vi "flip_switch.vi"(0 "PrepLineObject.lvclass":refnum<class "PrepLineObject.lvclass">, 3 "error in (no error)":errorcluster) -> (7 "PrepLineObject out":refnum<class "PrepLineObject.lvclass">, 10 "error out":errorcluster)   [LabVIEW 2017]
doc: "The switch that belongs to the \"PrepLineObject\" is being switched to the state as given in the private property."
uses:
  Classes/PrepLineObject/PrepLineObject.lvclass
  global variables.vi
  Classes/Instrument/instrument.lvclass
  Classes/StatusLog/StatusLog.lvclass
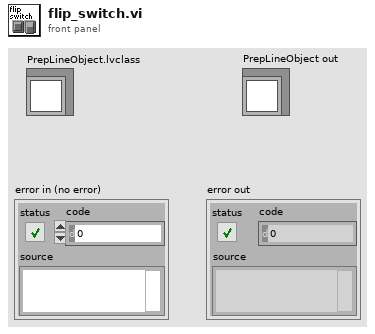
[diagram p1: front panel]
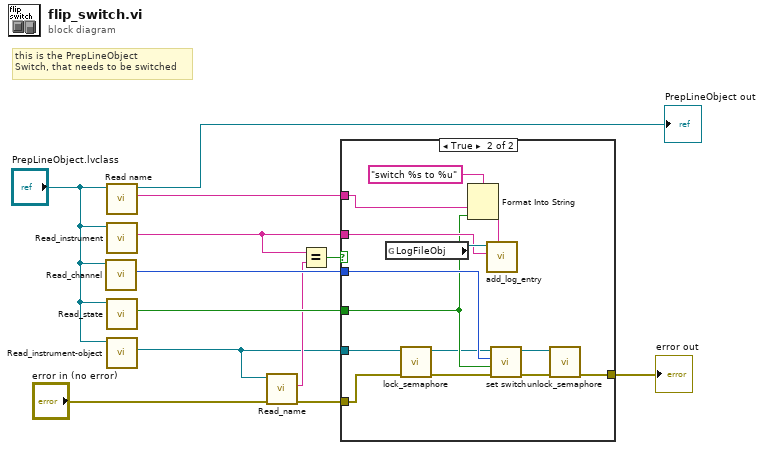
[diagram p0: block diagram]
diagram:
  # "this is the PrepLineObject\nSwitch, that needs to be switched"
  n1 = call-dynamic "Read_channel.vi"("PrepLineObject in"="PrepLineObject.lvclass") -> ("channel"=w7:u16)  [unwired: 8 in, 2 out]
  n2 = call-dynamic "Read name.vi"("PrepLineObject in"="PrepLineObject.lvclass") -> ("name"=w9:string, "PrepLineObject out"=→"PrepLineObject out":refnum<class "PrepLineObject.lvclass">)  [unwired: 8 in, 1 out]
  n3 = call-dynamic "Read_instrument.vi"("PrepLinePictureObjects in"="PrepLineObject.lvclass") -> ("instrument name"=w8:string)  [unwired: 7 in, 2 out]
  n4 = call-dynamic "Read_state.vi"("PrepLineObject in"="PrepLineObject.lvclass") -> ("state"=w6:bool)  [unwired: 8 in, 2 out]
  n5 = call-dynamic "Read_instrument-object.vi"("PrepLineObject in"="PrepLineObject.lvclass") -> ("instrument.lvclass"=w1:refnum<class "instrument.lvclass">)  [unwired: 8 in, 2 out]
  n6 = call-dynamic "Read_name.vi"("error in (no error)"="error in (no error)", "instrument in"=w1) -> ("error out"=w2:errorcluster, "name"=w4:string)  [unwired: 7 in, 1 out]
  n7 = Equal?(x=w8, y=w4) -> (x = y?=w3:bool)
  n8 = case shown="True" w3 {
    tunnel: w1 -> [_ w20]
    tunnel: w7 -> [_ w27]
    tunnel: w6 -> [_ w21]
    tunnel: w2 -> [w13 w19]
    tunnel: [w13 w14] -> w11
    tunnel: w9 -> [_ w22]
    tunnel: w8 -> [_ w23]
    frame False {
      # "wrong instrument"
    }
    frame True {
      n9 = global read "global variables.vi" "LogFileObj"() -> (w26:refnum<class "StatusLog.lvclass">)
      n10 = call-dynamic "lock_semaphore.vi"("error in (no error)"=w19, "instrument in"=w20) -> ("error out"=w17:errorcluster, "instrument out"=w18:refnum<class "instrument.lvclass">)  [unwired: 8 in]
      n11 = Format Into String(format string="switch %s to %u", w22, w21) -> (resulting string=w25:string)  [unwired: 2 in, 1 out]
      n12 = call-dynamic "add_log_entry.vi"("new entry"=w25, "log identifiers"=w23, "StatusLog in"=w26) -> ()  [unwired: 5 in, 2 out]
      n13 = call-dynamic "set switch.vi"("error in (no error)"=w17, "state"=w21, "channel"=w27, "instrument in"=w18) -> ("error out"=w15:errorcluster, "instrument out"=w16:refnum<class "instrument.lvclass">)  [unwired: 6 in]
      n14 = call-dynamic "unlock_semaphore.vi"("error in (no error)"=w15, "instrument in"=w16) -> ("error out"=w14:errorcluster)  [unwired: 8 in, 1 out]
    }
  }
  "error out" <- w11
